vi "Read message of the file header.vi"(8 "error in (no error)":errorcluster, 11 "Log File in":refnum<class "Events Log File.lvclass">) -> (0 "error out":errorcluster, 2 "message of the file header":string="----------------\nLOG FILE OF ACS\n----------------\n\nThis is the log file of ACS.  In this file, the messages generated during the execution of the softrware,\nas well as the commands received from the Graphical User Interface of SPARC4 are logged. ", 3 "Log File out":refnum<class "Events Log File.lvclass">)   [LabVIEW 2018, in "Events Log File.lvclass"]
uses:
  Events Log File.lvclass
  Events Log File.lvclass/Events Log File.ctl
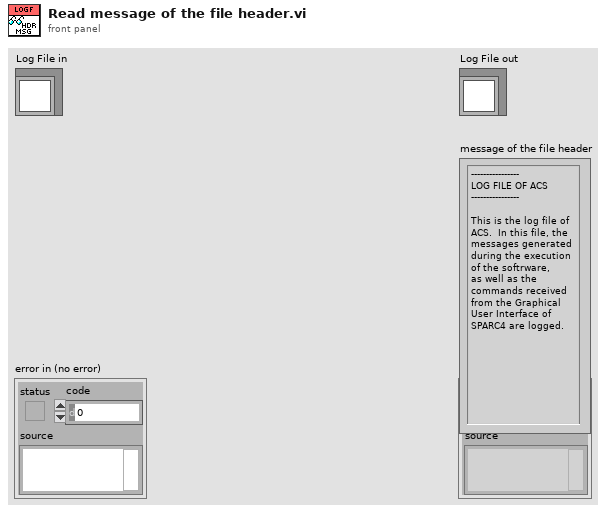
[diagram p1: front panel]
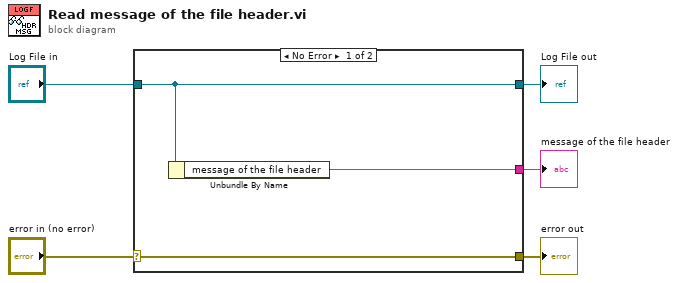
[diagram p0: block diagram]
diagram:
  n1 = case shown="No Error" "error in (no error)" {
    selector: "error in (no error)" -> [w8 w9]
    tunnel: [w8 w9] -> w4
    tunnel: [w7 w10] -> w2
    tunnel: "Log File in" -> [w7 w10]
    tunnel: [w6 _] -> w1
    frame No Error {
      n2 = Unbundle By Name(w7) -> ("message of the file header"=w6:string)
    }
    frame Error {
    }
  }
  "error out" <- w4
  "Log File out" <- w2
  "message of the file header" <- w1
